vi "Acquire from oscilloscope example.vi"() -> ()   [LabVIEW 2020]
doc: "This example shows how to use autosetup and acquire a waveform on a single channel."
uses:
  <vilib>/Analysis/baseanly.llb/Mean (DBL).vi
  <instrlib>/Tektronix TDS 200 1000 2000 Series/Public/Configure/Configure Trigger (Edge).vi
  <instrlib>/Tektronix TDS 200 1000 2000 Series/Tektronix TDS 200 1000 2000 Series.lvlib
  <vilib>/Analysis/NI_AALBase.lvlib
panel:
  out "Waveform Chart":dbl(graph)
  out "Waveform Graph":dbl[](graph)
  in  "Source (0: Channel 1)":u16(ring) items=["Channel 1", "Channel 2", "Channel 3", "Channel 4", "Math", "Reference A", "Reference B", "Reference C", "Reference D"]
  in  "Serial Configuration":T1={"Baud Rate"=9600, "Parity"=0, "Stop Bits"=10, "Flow Control"=2} {"Flow Control" items=["None", "XON/XOFF", "RTS/CTS", "XON/XOFF & RTS/CTS", "DTR/DSR", "XON/XOFF & DTR/DSR"]; "Stop Bits" items=["1.0"=10, "1.5"=15, "2.0"=20]; "Parity" items=["None", "Odd", "Even", "Mark", "Space"]; "Baud Rate" items=["300"=300, "600"=600, "1200"=1200, "2400"=2400, "4800"=4800, "9600"=9600, "19200"=19200]}
  in  "stop":bool
  in  "Timeout (10000 ms)":u32=10000
  in  "VISA resource name":refnum<visa-resource-name>
  # "(C) 2009-2015 National Instruments.  ALL RIGHTS RESERVED."
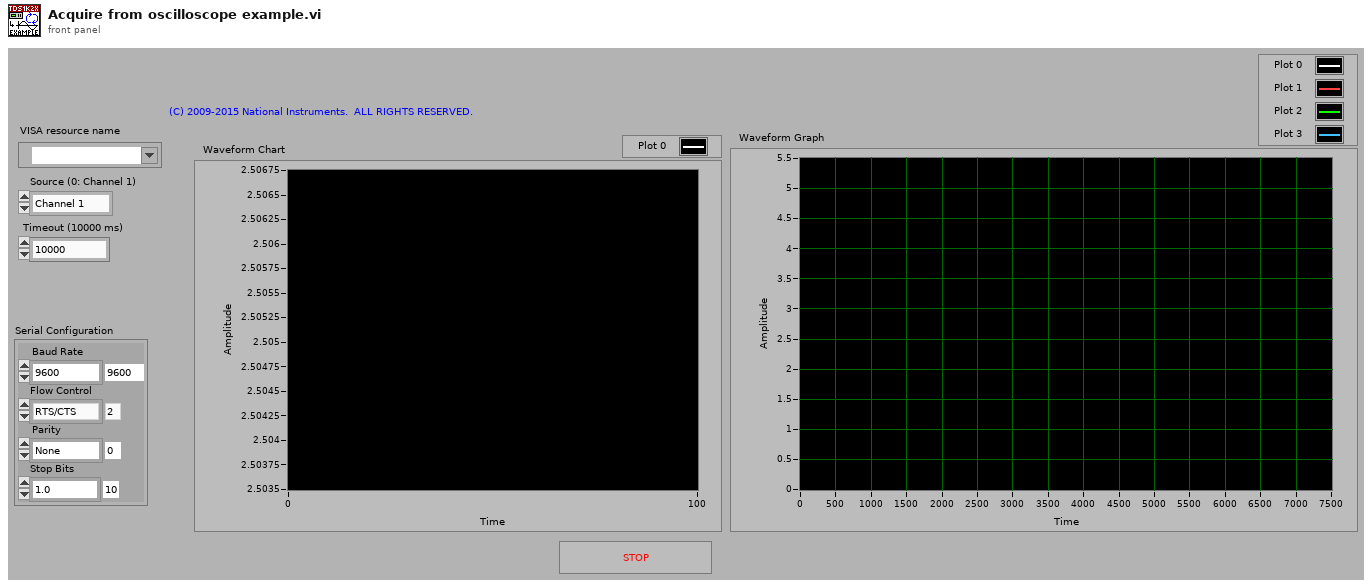
[diagram p1: front panel]
types:
  T1 = cluster{"Baud Rate":u32, "Parity":u16, "Stop Bits":u16, "Flow Control":u16}
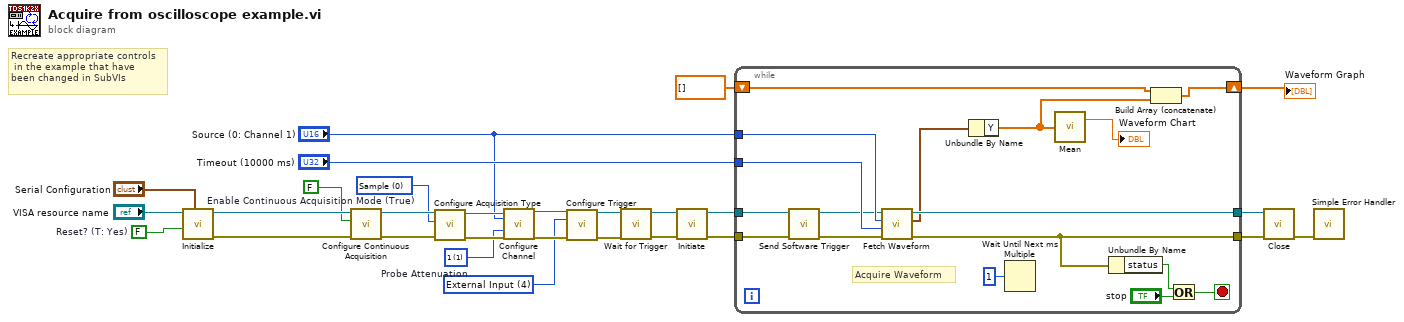
[diagram p0: block diagram]
diagram:
  w1 = 4 items=["Channel 1", "Channel 2", "Channel 3", "Channel 4", "External Input", "Attenuated External Input"] ("Trigger Source (0: Channel 1)")
  w8 = 1 items=["1"=1, "10"=10, "20"=20, "50"=50, "100"=100, "500"=500, "1000"=1000]  # Probe Attenuation
  w12 = 0 items=["Sample", "Average", "Peak Detect"] ("Acquisition Type (0: Sample)")
  w15 = FALSE  # Reset? (T: Yes)
  w20 = FALSE  # Enable Continuous Acquisition Mode (True)
  # "Recreate appropriate controls\n in the example that have \nbeen changed in SubVIs"
  n1 = call <instrlib>:"Initialize.vi"("Serial Configuration"="Serial Configuration", "Reset? (T: Yes)"=w15, "VISA resource name"="VISA resource name") -> ("error out"=w23:errorcluster, "VISA resource name out"=w22:refnum<visa-resource-name>)  [unwired: 2 in, 5 out]
  n2 = call <instrlib>:"Configure Continuous Acquisition.vi"("error in (no error)"=w23, "Enable Continuous Acquisition Mode (True)"=w20, "VISA resource name"=w22) -> ("error out"=w14:errorcluster, "VISA resource name out"=w13:refnum<visa-resource-name>)  [unwired: 7 out]
  n3 = call <instrlib>:"Configure Acquisition Type.vi"("error in (no error)"=w14, "Acquisition Type (0: Sample)"=w12, "VISA resource name"=w13) -> ("error out"=w10:errorcluster, "VISA resource name out"=w11:refnum<visa-resource-name>)  [unwired: 7 in]
  n4 = call <instrlib>:"Configure Channel.vi"("VISA resource name"=w11, "Channel (0: Channel 1)"="Source (0: Channel 1)", "Probe Attenuation (10: 10X)"=w8, "error in (no error)"=w10) -> ("VISA resource name out"=w5:refnum<visa-resource-name>, "error out"=w4:errorcluster)  [unwired: 10 in]
  n5 = call-poly <instrlib>:"Configure Trigger.vi"("VISA resource name"=w5, "Trigger Source (0: Channel 1)"=w1, "error in (no error)"=w4) -> ("VISA resource name out"=w2:refnum<visa-resource-name>, "error out"=w3:errorcluster)  [unwired: 11 in]
  n6 = call <instrlib>:"Wait for Trigger.vi"("error in (no error)"=w3, "VISA resource name"=w2) -> ("error out"=w6:errorcluster, "VISA resource name out"=w7:refnum<visa-resource-name>)  [unwired: 8 in]
  n7 = call <instrlib>:"Initiate.vi"("error in (no error)"=w6, "VISA resource name"=w7) -> ("error out"=w18:errorcluster, "VISA resource name out"=w19:refnum<visa-resource-name>)  [unwired: 8 out]
  n8 = while {
    tunnel: w19 -> [w34]
    tunnel: w18 -> [w32]
    tunnel: [w38] -> w27
    tunnel: [w39] -> w26
    tunnel: "Timeout (10000 ms)" -> [w45]
    tunnel: "Source (0: Channel 1)" -> [w40]
    shift-right: [w36] -> w17
    shift-left: dbl[] [] -> [w37]
    stop <- w43 stop-if-true
    # "Acquire Waveform"
    n9 = call <instrlib>:"Send Software Trigger.vi"("error in (no error)"=w32, "VISA resource name"=w34) -> ("error out"=w31:errorcluster, "VISA resource name out"=w33:refnum<visa-resource-name>)  [unwired: 8 in]
    n10 = call <instrlib>:"Fetch Waveform.vi"("error in (no error)"=w31, "Timeout (10000 ms)"=w45, "Source (0: Channel 1)"=w40, "VISA resource name"=w33) -> ("error out"=w39:errorcluster, "Waveform Data"=w35:waveform(dbl), "VISA resource name out"=w38:refnum<visa-resource-name>)  [unwired: 5 out]
    n11 = Unbundle By Name(w35) -> ("Y"=w30:dbl[])
    n12 = Wait Until Next ms Multiple(millisecond multiple=u32 1) -> ()  [unwired: 1 out]
    n13 = call-poly <vilib>:"Mean.vi"("X"=w30) -> ("mean"=→"Waveform Chart":dbl)  [unwired: 1 out]
    n14 = Unbundle By Name(w39) -> ("status"=w42:bool)
    n15 = Build Array (concatenate)(w37, w30) -> (w36:dbl[])
    n16 = Or(x=w42, y="stop") -> (x .or. y?=w43:bool)
  }
  "Waveform Graph" <- w17
  n17 = call <instrlib>:"Close.vi"("error in (no error)"=w26, "VISA resource name"=w27) -> ("error out"=w28:errorcluster)  [unwired: 9 out]
  n18 = call <vilib>:"Simple Error Handler.vi"("error in (no error)"=w28) -> ()  [unwired: 1 in, 8 out]
